vi "get_paths.vi"(5 "settings file name (without ending)":string, 7 "configuration file name (without ending)":string, 8 "error in (no error)":errorcluster, 9 "component name":string, 10 "component type":string, 11 "user":string) -> (0 "error out":errorcluster, 1 "settings paths":T3, 2 "configuration paths":T2, 3 "component paths":T1={"components directory"=path "C:/helioscan/components", "component type directory"=path "", "specific component directory"=path "C:/helioscan/main/labview_source/type_definitions/classes/GenericComponent", "component class path"=path "C:/helioscan/main/labview_source/type_definitions/classes/GenericComponent/GenericComponent.lvclass"})   [LabVIEW 2010]
uses:
  clusters/settings_paths_cluster.ctl
  clusters/configuration_paths_cluster.ctl
  classes/GenericComponent/GenericComponent/component_path_clusters.ctl
panel:
  # "(e.g., C:\\helioscan\\components\\Stage\\StageDL090602SutterMP285\\StageDL090602SutterMP285\\StageDL090602SutterMP285.lvclass)"
  # "(e.g., C:\\helioscan\\components\\Stage\\StageDL090602SutterMP285\\StageDL090602SutterMP285\\)"
  # "(e.g., C:\\helioscan\\components\\Stage)"
  # "(e.g., C:\\helioscan\\components)"
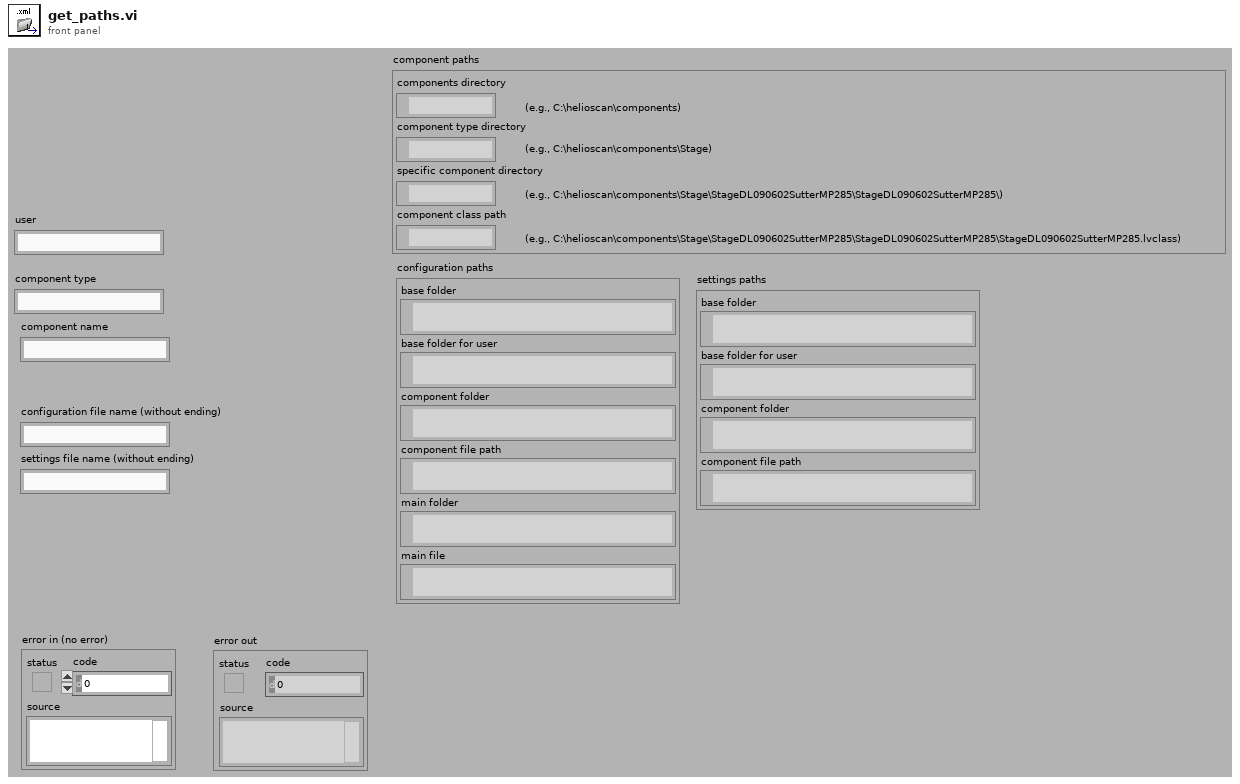
[diagram p1: front panel]
types:
  T1 = typedef "component_path_clusters.ctl" = cluster{"components directory":path, "component type directory":path, "specific component directory":path, "component class path":path}
  T2 = typedef "configuration_paths_cluster.ctl" = cluster{"base folder":path, "base folder for user":path, "component folder":path, "component file path":path, "main folder":path, "main file":path}
  T3 = typedef "settings_paths_cluster.ctl" = cluster{"base folder":path, "base folder for user":path, "component folder":path, "component file path":path}
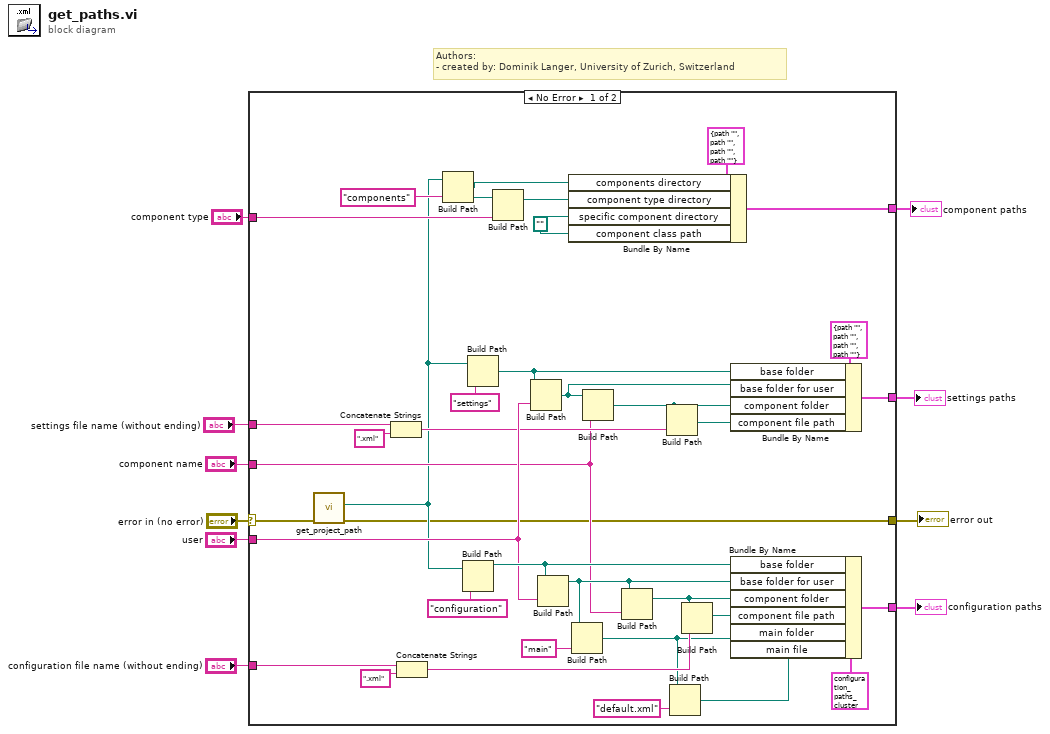
[diagram p0: block diagram]
diagram:
  # "Authors: \n- created by: Dominik Langer, University of Zurich, Switzerland"
  n1 = case shown="No Error" "error in (no error)" {
    selector: "error in (no error)" -> [w12 w47]
    tunnel: [w11 w47] -> w5
    tunnel: [w38 _] -> w7
    tunnel: [w41 _] -> w6
    tunnel: "settings file name (without ending)" -> [w30 _]
    tunnel: [w25 _] -> w3
    tunnel: "component type" -> [w24 _]
    tunnel: "user" -> [w23 _]
    tunnel: "component name" -> [w21 _]
    tunnel: "configuration file name (without ending)" -> [w19 _]
    frame No Error {
      w20 = path ""
      n2 = call "get_project_path.vi"("error in (no error)"=w12) -> ("error out"=w11:errorcluster, "helioscan path"=w13:path)  [unwired: 9 in]
      n3 = Concatenate Strings(w30, ".xml" ("string")) -> (w22:string)
      n4 = Concatenate Strings(w19, ".xml" ("string")) -> (w17:string)
      n5 = Build Path(base path=w13, name or relative path="components") -> (appended path=w27:path)
      n6 = Build Path(base path=w13, name or relative path="configuration") -> (appended path=w37:path)
      n7 = Build Path(base path=w13, name or relative path="settings") -> (appended path=w44:path)
      n8 = Build Path(base path=w27, name or relative path=w24) -> (appended path=w26:path)
      n9 = Build Path(base path=w44, name or relative path=w23) -> (appended path=w34:path)
      n10 = Build Path(base path=w37, name or relative path=w23) -> (appended path=w32:path)
      n11 = Bundle By Name(cluster=T1 {"components directory"=path "", "component type directory"=path "", "specific component directory"=path "", "component class path"=path ""} ("component paths"), "components directory"=w27, "component type directory"=w26, "specific component directory"=w20, "component class path"=w20) -> (w25:T1)
      n12 = Build Path(base path=w32, name or relative path="main") -> (appended path=w16:path)
      n13 = Build Path(base path=w34, name or relative path=w21) -> (appended path=w43:path)
      n14 = Build Path(base path=w32, name or relative path=w21) -> (appended path=w35:path)
      n15 = Build Path(base path=w43, name or relative path=w22) -> (appended path=w42:path)
      n16 = Build Path(base path=w16, name or relative path="default.xml") -> (appended path=w15:path)
      n17 = Build Path(base path=w35, name or relative path=w17) -> (appended path=w36:path)
      n18 = Bundle By Name(cluster=T3 {"base folder"=path "", "base folder for user"=path "", "component folder"=path "", "component file path"=path ""} ("settings paths"), "base folder"=w44, "base folder for user"=w34, "component folder"=w43, "component file path"=w42) -> (w41:T3)
      n19 = Bundle By Name(cluster=T2 {"base folder"=path "", "base folder for user"=path "", "component folder"=path "", "component file path"=path "", "main folder"=path "", "main file"=path ""} ("configuration paths"), "base folder"=w37, "base folder for user"=w32, "component folder"=w35, "component file path"=w36, "main folder"=w16, "main file"=w15) -> (w38:T2)
    }
    frame Error {
    }
  }
  "error out" <- w5
  "settings paths" <- w6
  "configuration paths" <- w7
  "component paths" <- w3
